vi "run2.vi"   [LabVIEW 2016, in "LineFollower2Sensor.lvrbt"]
uses:
  LineFollower2Sensor.lvrbt
  <vilib>/NXT/Hardware/Plugins/Tetrix DC Motor/TetrixDCMotorAddress.ctl
  <vilib>/NXT/Block Support/NXT_InputPort.ctl
  <vilib>/NXT/NXTIO Xnodes/NXTIONodeSubVIs/TETRIX IO Move DC Motors.vi
  <vilib>/NXT/Dual Mode Library/Sensors/EV3_Color_Reflect.vi
  <vilib>/NXT/Subs/LVHSConnector.ctl
  <vilib>/NXT/NXTIO Xnodes/AddressXNode/NXTIOAddress.xnode
  <vilib>/NXT/NXTIO Xnodes/NXTIOXNode/NXTIO.xnode
  <vilib>/NXT/LegoClasses/BrickReference/BrickReference.lvclass
types:
  T1 = typedef "TetrixDCMotorAddress.ctl" = i32
  T2 = typedef "LVHSConnector.ctl" = refnum<class "BrickReference.lvclass">
  T3 = cluster{"TetrixDCMotor":T1, "TetrixDCMotor 2":T1}
  T4 = typedef "NXT_InputPort.ctl" = u32
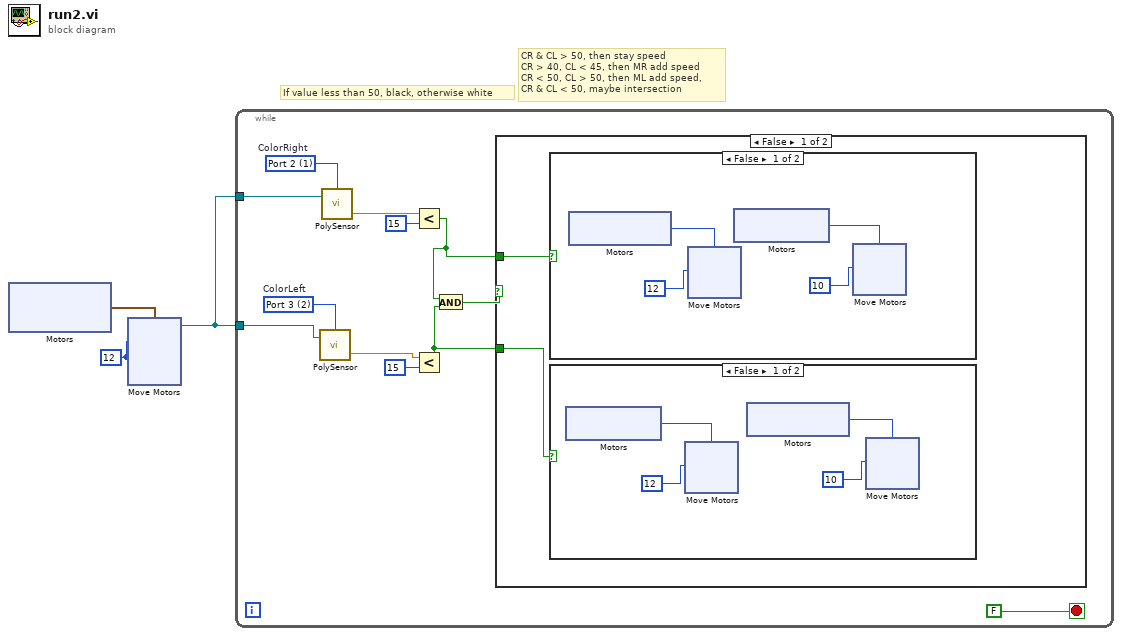
[diagram p0: block diagram]
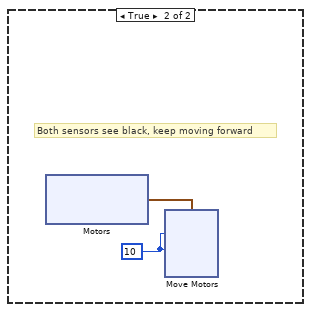
[diagram p4: hidden frame]
diagram:
  w3 = i8 12 ("Power/Speed 2")
  # "CR & CL > 50, then stay speed\nCR > 40, CL < 45, then MR add speed\nCR < 50, CL > 50, then ML add speed,\nCR & CL < 50, maybe intersection"
  # "If value less than 50, black, otherwise white"
  n1 = xnode "Motors"() -> ("Motor"=w2:cluster{"TetrixDCMotor":T1, "TetrixDCMotor":T1})
  n2 = xnode "Move Motors"("Power/Speed 2"=w3, "Power/Speed 1"=w3, "Motors"=w2) -> ("NXT/EV3"=w1:T2)  [unwired: 1 in]
  n3 = while {
    tunnel: w1 -> [w5]
    tunnel: w1 -> [w4]
    stop <- FALSE stop-if-true
    w13 = T4 2 items=["Port 1", "Port 2", "Port 3", "Port 4"]  # ColorLeft
    w14 = T4 1 items=["Port 1", "Port 2", "Port 3", "Port 4"]  # ColorRight
    n4 = call-poly <vilib>:"PolySensor.vi"("NXT/EV3"=w4, "Port (Port 1)"=w13) -> ("Scaled Value"=w9:sgl)  [unwired: 1 in, 1 out]
    n5 = call-poly <vilib>:"PolySensor.vi"("NXT/EV3"=w5, "Port (Port 1)"=w14) -> ("Scaled Value"=w12:sgl)  [unwired: 1 in, 1 out]
    n6 = Less?(x=w12, y=i16 15) -> (x < y?=w7:bool)
    n7 = Less?(x=w9, y=i16 15) -> (x < y?=w6:bool)
    n8 = And(x=w7, y=w6) -> (x .and. y?=w8:bool)
    n9 = case "Case 1 and 4" shown="False" w8 {
      tunnel: w7 -> [w17 _]
      tunnel: w6 -> [w16 _]
      frame False {
        n10 = case shown="False" w17 {
          frame False {
            n11 = xnode "Motors"() -> ("Motor"=w40:T1)
            n12 = xnode "Move Motors"("Power/Speed 1"=i8 12 ("Power/Speed 2"), "Motors"=w40) -> ()  [unwired: 1 in, 1 out]
            n13 = xnode "Motors"() -> ("Motor"=w38:T1)
            n14 = xnode "Move Motors"("Power/Speed 1"=i8 10 ("Power/Speed 2"), "Motors"=w38) -> ()  [unwired: 1 in, 1 out]
          }
          frame True {
          }
        }
        n15 = case shown="False" w16 {
          frame False {
            n16 = xnode "Motors"() -> ("Motor"=w21:T1)
            n17 = xnode "Move Motors"("Power/Speed 1"=i8 12 ("Power/Speed 2"), "Motors"=w21) -> ()  [unwired: 1 in, 1 out]
            n18 = xnode "Motors"() -> ("Motor"=w19:T1)
            n19 = xnode "Move Motors"("Power/Speed 1"=i8 10 ("Power/Speed 2"), "Motors"=w19) -> ()  [unwired: 1 in, 1 out]
          }
          frame True {
          }
        }
      }
      frame True {
        w58 = i8 10 ("Power/Speed 2")
        # "Both sensors see black, keep moving forward"
        n20 = xnode "Motors"() -> ("Motor"=w59:cluster{"TetrixDCMotor":T1, "TetrixDCMotor":T1})
        n21 = xnode "Move Motors"("Power/Speed 2"=w58, "Power/Speed 1"=w58, "Motors"=w59) -> ()  [unwired: 1 in, 1 out]
      }
    }
  }
